vi "setJustification.vi"(0 "reference":refnum<class "MultiLineString.lvclass">, 1 "justification":T1, 5 "error in (no error)":errorcluster) -> (14 "reference out":refnum<class "MultiLineString.lvclass">, 19 "error out":errorcluster)   [LabVIEW 2016, in "MultiLineString.lvclass"]
doc: "public void setJustification(int newValue)"
uses:
  <resource>/Framework/Providers/Open_GDS/UML/MultiLineString_class/MultiLineString.lvclass
  <resource>/Framework/Providers/Open_GDS/UML/MultiLineString_class/JustificationType.ctl
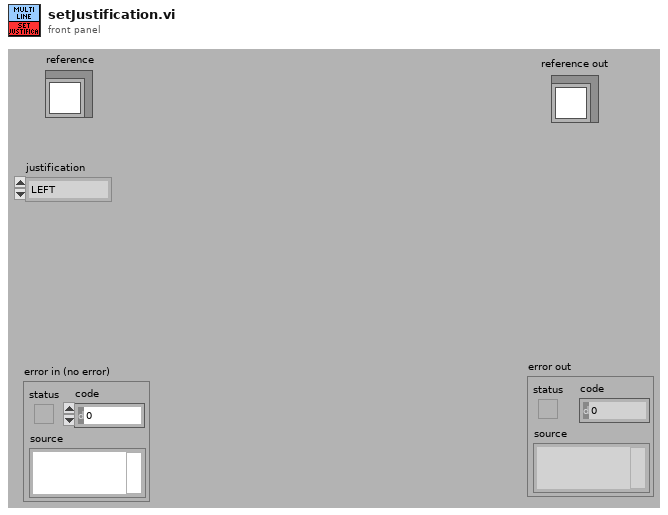
[diagram p1: front panel]
types:
  T1 = typedef "MultiLineString.lvclass/JustificationType.ctl" = enum16{"LEFT", "CENTER", "RIGHT"}
  T2 = typedef "MultiLineString.lvclass/ObjectAttributes.ctl" = cluster{"GAP":i32, "text":string, "justification":T1, "size":T3, "underlined":bool}
  T3 = typedef "MultiLineString.lvclass/SizeType.ctl" = enum16{"LARGE", "NORMAL", "SMALL"}
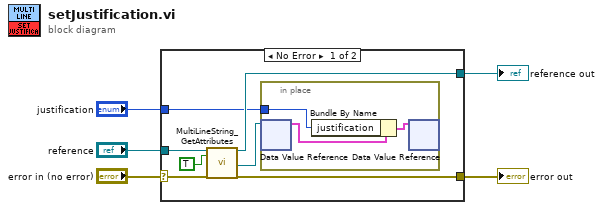
[diagram p0: block diagram]
diagram:
  n1 = case shown="No Error" "error in (no error)" {
    selector: "error in (no error)" -> [w12 w16]
    tunnel: "reference" -> [w11 w17]
    tunnel: [w10 w16] -> w3
    tunnel: [w9 w17] -> w2
    tunnel: "justification" -> [w6 _]
    frame No Error {
      n2 = call <resource>:"MultiLineString_GetAttributes.vi"("reference in"=w11, "OnlyGetDvrReference(False)"=TRUE, "error in (no error)"=w12) -> ("reference out"=w9:refnum<class "MultiLineString.lvclass">, "DataRef"=w7:refnum<data-value>, "error out"=w10:errorcluster)  [unwired: 13 in, 1 out]
      n3 = in-place {
        in-place-border: w6 -> [w14]
        n4 = in-place-dvr #1(w7) -> (w15:T2)  [unwired: 1 out]
        n5 = Bundle By Name(cluster=w15, "justification"=w14) -> (w13:T2)
        n6 = in-place-dvr #1(w13) -> ()  [unwired: 2 out]
      }
    }
    frame Error {
    }
  }
  "reference out" <- w2
  "error out" <- w3
